vi "ExecuteSpeed.vi"(8 "Error In":errorcluster, 11 "RobotDriveDevRef":T1={"DevStatus"={"status"=FALSE, "code"=0, "source"=""}, "Motors[]"=[], "Square Inputs"=FALSE, "Max Output"=1.0}) -> (0 "Error Out":errorcluster)   [LabVIEW 2020]
uses:
  <vilib>/Rock Robotics/WPI/RobotDrive/WPI_RobotDriveDevRef.ctl
  <vilib>/Rock Robotics/WPI/MotorControl/WPI_MotorControlDeviceRef.ctl
  <vilib>/Rock Robotics/WPI/MotorControl/WPI_MotorControlType.ctl
  <vilib>/Rock Robotics/SystemInterfaces/DIO/FPGA_DIOPWMChannel.ctl
  <vilib>/Rock Robotics/WPI/PWM/WPI_PWMDeadband.ctl
  <vilib>/Rock Robotics/SystemInterfaces/DIO/FPGA_DIOChannel.ctl
  <vilib>/Rock Robotics/WPI/ThirdParty/JAS_Junk/TrajLib/SlewRateLimiter_New.vi
  <vilib>/Rock Robotics/WPI/ThirdParty/JAS_Junk/TrajLib/SlewRateLimiter_Reset.vi
  <vilib>/Rock Robotics/WPI/ThirdParty/JAS_Junk/TrajLib/SlewRateLimiter_Calculate.vi
  <vilib>/Rock Robotics/WPI/ThirdParty/JAS_Junk/TrajLib/SlewRateLimiter_SetRate.vi
  <vilib>/Rock Robotics/WPI/ThirdParty/JAS_Junk/TrajLib/PIDController_AtSetpoint.vi
  <vilib>/Rock Robotics/WPI/ThirdParty/JAS_Junk/TrajLib/PIDController_SetPIDF.vi
  <vilib>/Rock Robotics/WPI/ThirdParty/JAS_Junk/TrajLib/PIDController_SetDerivativeFilter.vi
  <vilib>/Rock Robotics/WPI/ThirdParty/JAS_Junk/TrajLib/PIDController_SetIntegratorRange.vi
  <vilib>/Rock Robotics/WPI/ThirdParty/JAS_Junk/TrajLib/PIDController_SetTolerancePandV.vi
  <vilib>/Rock Robotics/WPI/ThirdParty/JAS_Junk/TrajLib/PIDController_DisableContinousInput.vi
  <vilib>/Rock Robotics/WPI/ThirdParty/JAS_Junk/TrajLib/PIDController_EnableContinousInput.vi
  <vilib>/Rock Robotics/WPI/ThirdParty/JAS_Junk/TrajLib/PIDController_Reset.vi
  <vilib>/Rock Robotics/WPI/ThirdParty/JAS_Junk/TrajLib/PIDController_New.vi
  <vilib>/Rock Robotics/WPI/ThirdParty/JAS_Junk/TrajLib/PIDController_SetOutputLimits.vi
  <vilib>/Rock Robotics/WPI/ThirdParty/JAS_Junk/TrajLib/ControllerUtil_GetModulusError.vi
  <vilib>/Rock Robotics/WPI/ThirdParty/JAS_Junk/TrajLib/PIDController_NewPeriod.vi
  <vilib>/Rock Robotics/SystemInterfaces/NetworkCommunication/NetComm_UsageReport_report.vi
  DriveGlobals.vi
  <vilib>/Rock Robotics/WPI/ThirdParty/JAS_Junk/TrajLib/Util_GetTime.vi
  <vilib>/Rock Robotics/WPI/ThirdParty/JAS_Junk/TrajLib/Util_LibraryGlobals.vi
  <vilib>/Rock Robotics/WPI/ThirdParty/JAS_Junk/TrajLib/PIDController_AdvCalculate_FF_Sp_Pv.vi
  <vilib>/Rock Robotics/Network Tables/NT Write Numeric Array.vi
  <vilib>/Rock Robotics/WPI/ThirdParty/JAS_Junk/TrajLib/Trajectory_Library.lvlib
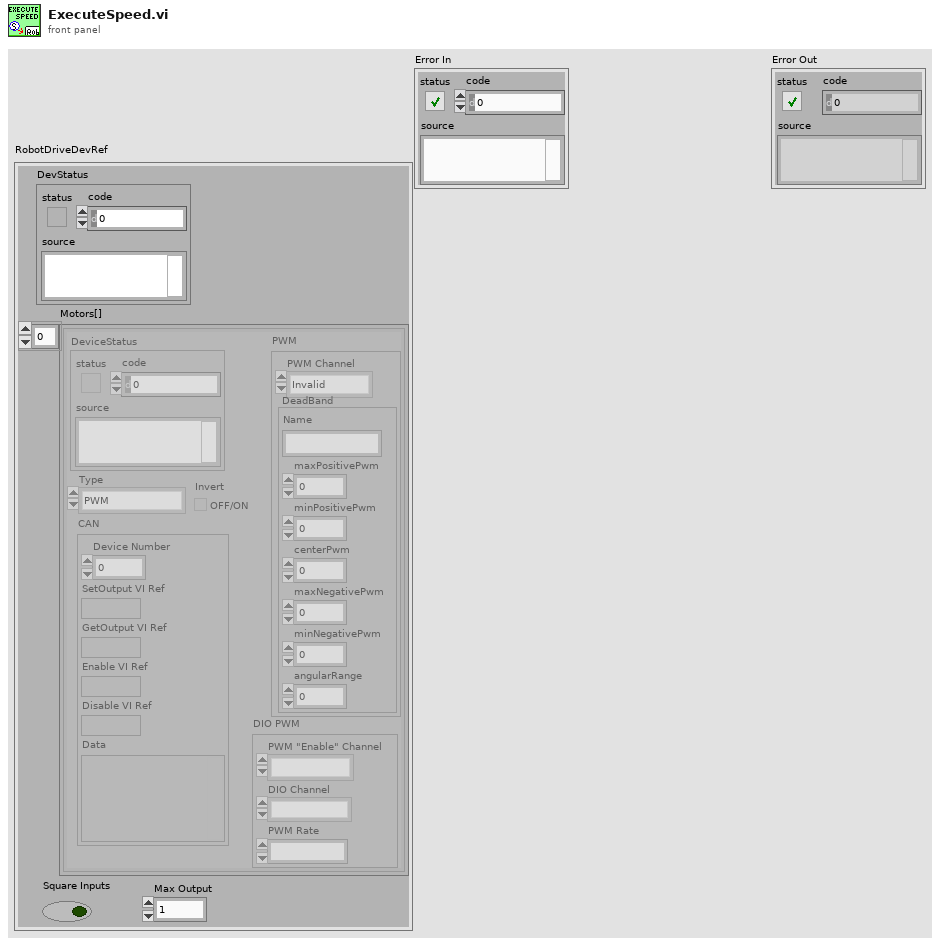
[diagram p1: front panel]
types:
  T1 = typedef "WPI_RobotDriveDevRef.ctl" = cluster{"DevStatus":errorcluster, "Motors[]":T2[], "Square Inputs":bool, "Max Output":dbl}
  T2 = typedef "WPI_MotorControlDeviceRef.ctl" = cluster{"DeviceStatus":errorcluster, "Type":T3, "PWM":cluster{"PWM Channel":T4, "DeadBand":T5}, "CAN":cluster{"Device Number":u8, "SetOutput VI Ref":variant, "GetOutput VI Ref":variant, "Enable VI Ref":variant, "Disable VI Ref":variant, "Data":variant}, "Invert":bool, "DIO PWM":cluster{"PWM \"Enable\" Channel":T4, "DIOChannel":T6, "PWM Rate":dbl}}
  T3 = typedef "WPI_MotorControlType.ctl" = enum16{"PWM", "CAN", "DIO PWM"}
  T4 = typedef "FPGA_DIOPWMChannel.ctl" = enum8{"PWM 0", "PWM 1", "PWM 2", "PWM 3", "PWM 4", "PWM 5", "PWM 6", "PWM 7", "PWM 8", "PWM 9", "PWM MXP 0", "PWM MXP 1", "PWM MXP 2", "PWM MXP 3", "PWM MXP 4", "PWM MXP 5", "PWM MXP 6", "PWM MXP 7", "PWM MXP 8", "PWM MXP 9", "Invalid"}
  T5 = typedef "WPI_PWMDeadband.ctl" = cluster{"Name":string, "maxPositivePwm":i32, "minPositivePwm":i32, "centerPwm":i32, "maxNegativePwm":i32, "minNegativePwm":i32, "angularRange":u16}
  T6 = typedef "FPGA_DIOChannel.ctl" = enum8{"DIO 0", "DIO 1", "DIO 2", "DIO 3", "DIO 4", "DIO 5", "DIO 6", "DIO 7", "DIO 8", "DIO 9", "DIO MXP 0", "DIO MXP 1", "DIO MXP 2", "DIO MXP 3", "DIO MXP 4", "DIO MXP 5", "DIO MXP 6", "DIO MXP 7", "DIO MXP 8", "DIO MXP 9", "DIO MXP 10", "DIO MXP 11", "DIO MXP 12", "DIO MXP 13", "DIO MXP 14", "DIO MXP 15", "SPI Port CS1", "SPI Port CS2", "SPI Port CS3", "SPI Port MISO", "SPI Port MOSI", "Invalid"}
  T7 = typedef "Trajectory_Library.lvlib/PID_ADV_LIMITS.ctl" = cluster{"MaxInput":dbl, "MinInput":dbl, "Continuous":bool, "MaxOutput":dbl, "MinOutput":dbl}
  T8 = typedef "Trajectory_Library.lvlib/PID_ADV_TUNING.ctl" = cluster{"Kf":dbl, "Kp":dbl, "Ki":dbl, "Kd":dbl, "MaximumIntegral":dbl, "MinimumIntegral":dbl, "Filter Derivative":bool}
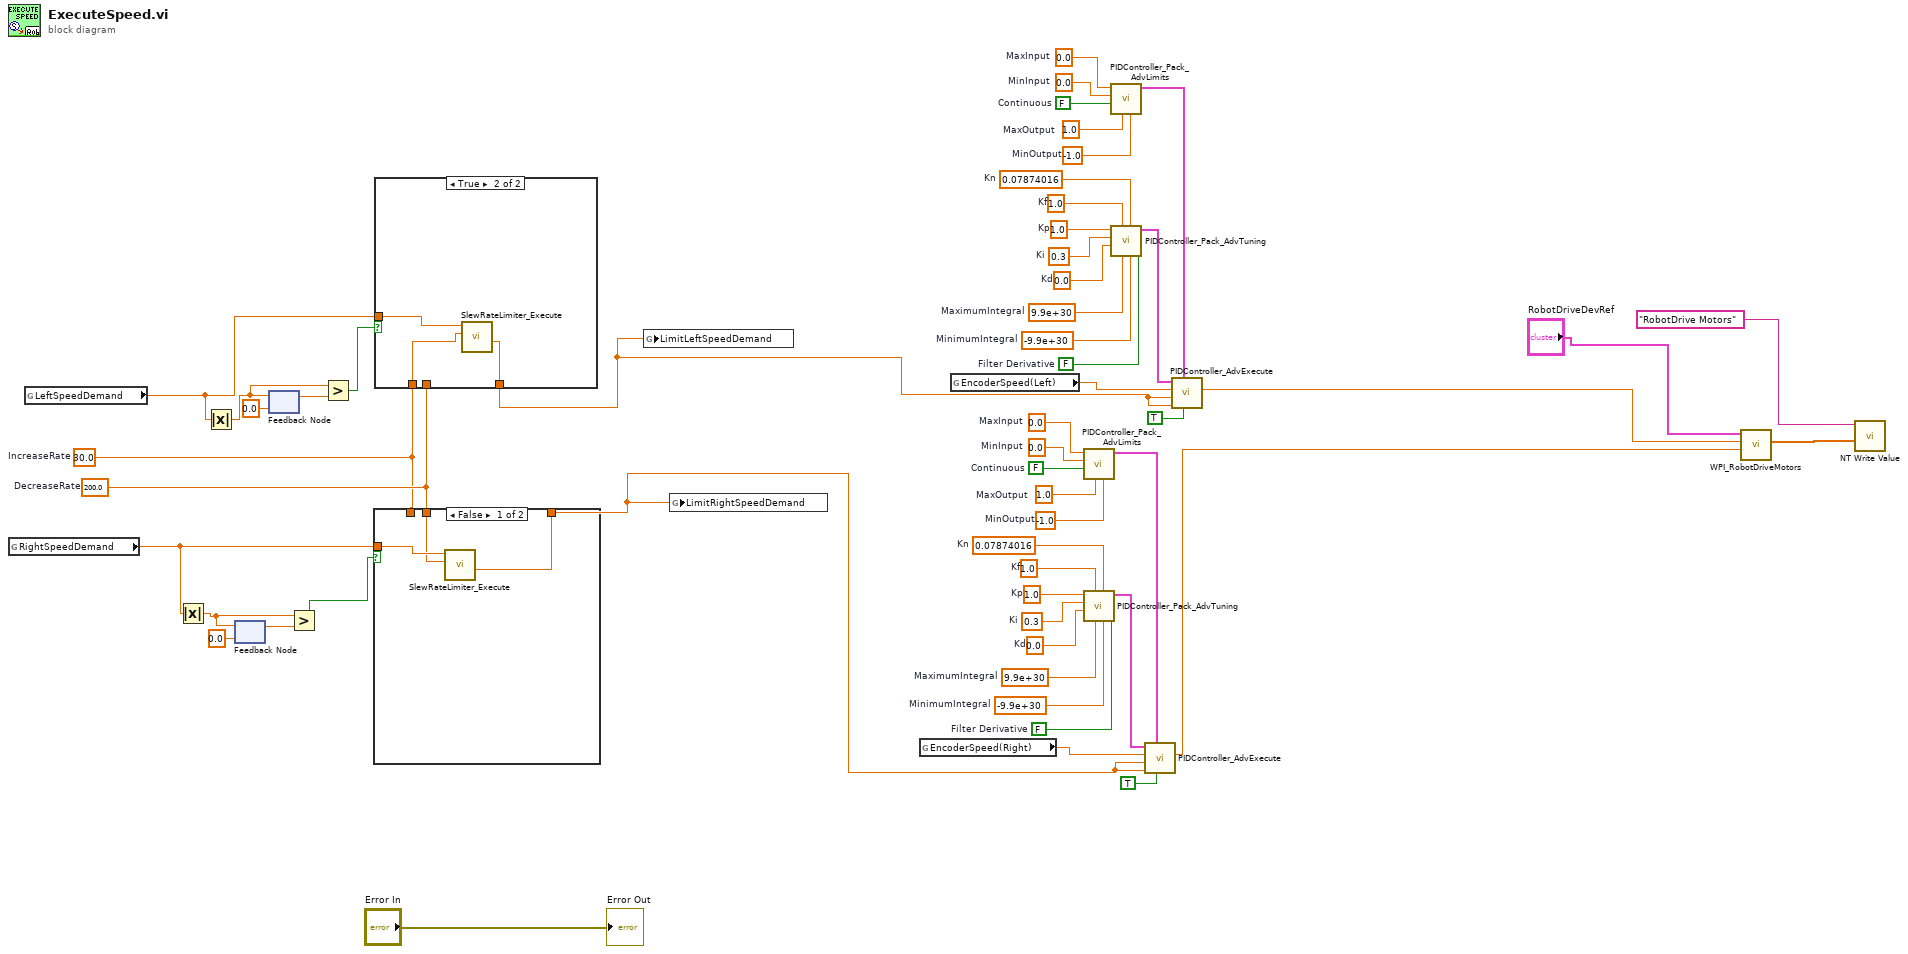
[diagram p0: block diagram]
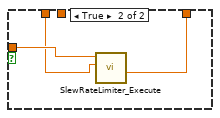
[diagram p2: hidden frame]
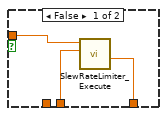
[diagram p3: hidden frame]
diagram:
  w27 = 0.07874016  # Kn
  w26 = 1.0  # Kp
  w25 = 0.3  # Ki
  w24 = 0.0  # Kd
  w23 = 1.0  # Kf
  w22 = 9.9e+30  # MaximumIntegral
  w21 = -9.9e+30  # MinimumIntegral
  w20 = FALSE  # Filter Derivative
  w18 = 0.0  # MinInput
  w17 = FALSE  # Continuous
  w16 = 1.0  # MaxOutput
  w19 = -1.0  # MinOutput
  w15 = 0.0  # MaxInput
  w44 = 0.07874016  # Kn
  w43 = 1.0  # Kp
  w42 = 0.3  # Ki
  w41 = 0.0  # Kd
  w40 = 1.0  # Kf
  w39 = 9.9e+30  # MaximumIntegral
  w38 = -9.9e+30  # MinimumIntegral
  w37 = FALSE  # Filter Derivative
  w35 = 0.0  # MinInput
  w34 = FALSE  # Continuous
  w33 = 1.0  # MaxOutput
  w36 = -1.0  # MinOutput
  w32 = 0.0  # MaxInput
  w46 = 200.0  # DecreaseRate
  w45 = 30.0  # IncreaseRate
  n1 = global read "DriveGlobals.vi" "RightSpeedDemand"() -> (w7:dbl)
  n2 = global read "DriveGlobals.vi" "LeftSpeedDemand"() -> (w5:dbl)
  n3 = Absolute Value(x=w7) -> (abs(x)=w8:dbl)
  n4 = Absolute Value(x=w5) -> (abs(x)=w6:dbl)
  n5 = feedback #1(0.0 ("LeftSpeedDemand")) -> (w48:dbl)
  n6 = feedback-in #1(w8) -> ()
  n7 = feedback-in #2(w6) -> ()
  n8 = feedback #2(0.0 ("LeftSpeedDemand")) -> (w51:dbl)
  n9 = Greater?(x=w8, y=w48) -> (0:w4:bool)
  n10 = Greater?(x=w6, y=w51) -> (0:w50:bool)
  n11 = case shown="False" w4 {
    tunnel: [w55 w58] -> w9
    tunnel: w7 -> [w57 w60]
    tunnel: w45 -> [_ w59]
    tunnel: w46 -> [w56 _]
    frame False {
      n12 = call <vilib>:"SlewRateLimiter_Execute.vi"("Rate"=w56, "Input"=w57) -> ("Output"=w55:dbl)  [unwired: 8 in, 1 out]
    }
    frame True {
      n13 = call <vilib>:"SlewRateLimiter_Execute.vi"("Rate"=w59, "Input"=w60) -> ("Output"=w58:dbl)  [unwired: 8 in, 1 out]
    }
  }
  n14 = case shown="True" w50 {
    tunnel: [w61 w64] -> w10
    tunnel: w5 -> [w63 w66]
    tunnel: w45 -> [_ w65]
    tunnel: w46 -> [w62 _]
    frame False {
      n15 = call <vilib>:"SlewRateLimiter_Execute.vi"("Rate"=w62, "Input"=w63) -> ("Output"=w61:dbl)  [unwired: 8 in, 1 out]
    }
    frame True {
      n16 = call <vilib>:"SlewRateLimiter_Execute.vi"("Rate"=w65, "Input"=w66) -> ("Output"=w64:dbl)  [unwired: 8 in, 1 out]
    }
  }
  n17 = global write "DriveGlobals.vi" "LimitLeftSpeedDemand"(w10) -> ()
  n18 = global write "DriveGlobals.vi" "LimitRightSpeedDemand"(w9) -> ()
  n19 = global read "DriveGlobals.vi" "EncoderSpeed(Right)"() -> (w28:dbl)
  n20 = global read "DriveGlobals.vi" "EncoderSpeed(Left)"() -> (w12:dbl)
  n21 = call <vilib>:"PIDController_Pack_AdvLimits.vi"("MinOutput"=w36, "MaxOutput"=w33, "Continuous"=w34, "MinInput"=w35, "MaxInput"=w32) -> ("Adv PID Limits"=w30:T7)  [unwired: 6 in]
  n22 = call <vilib>:"PIDController_Pack_AdvTuning.vi"("Filter Derivative"=w37, "MinimumIntegral"=w38, "Kn"=w44, "MaximumIntegral"=w39, "Kf"=w40, "Kd"=w41, "Ki"=w42, "Kp"=w43) -> ("Adv PID Tuning"=w31:T8)  [unwired: 3 in]
  n23 = call <vilib>:"PIDController_Pack_AdvLimits.vi"("MinOutput"=w19, "MaxOutput"=w16, "Continuous"=w17, "MinInput"=w18, "MaxInput"=w15) -> ("Adv PID Limits"=w13:T7)  [unwired: 6 in]
  n24 = call <vilib>:"PIDController_Pack_AdvTuning.vi"("Filter Derivative"=w20, "MinimumIntegral"=w21, "Kn"=w27, "MaximumIntegral"=w22, "Kf"=w23, "Kd"=w24, "Ki"=w25, "Kp"=w26) -> ("Adv PID Tuning"=w14:T8)  [unwired: 3 in]
  n25 = call <vilib>:"PIDController_AdvExecute.vi"("Auto"=TRUE, "Adv PID Limits"=w30, "FF-FeedForward"=w9, "SP-SetPoint"=w9, "PV-Measurement"=w28, "Adv PID Tuning"=w31) -> ("CO-ControlOutput"=w29:dbl)  [unwired: 3 in, 2 out]
  n26 = call <vilib>:"PIDController_AdvExecute.vi"("Auto"=TRUE, "Adv PID Limits"=w13, "FF-FeedForward"=w10, "SP-SetPoint"=w10, "PV-Measurement"=w12, "Adv PID Tuning"=w14) -> ("CO-ControlOutput"=w11:dbl)  [unwired: 3 in, 2 out]
  n27 = call <vilib>:"WPI_RobotDriveMotors.vi"("RightSpeed"=w29, "LeftSpeed"=w11, "RobotDriveDevRef"="RobotDriveDevRef") -> ("Motor Values"=w54:dbl[])  [unwired: 6 in, 2 out]
  n28 = call-poly <vilib>:"NT Write Value.vi"("Numeric Array"=w54, "Name"="RobotDrive Motors") -> ()  [unwired: 9 in, 1 out]
  "Error Out" <- "Error In"
